vi "sub_PSKMod.vi"(0 "Packet to Transmit":i8[](array[numeric]), 2 "PSK system parameters":T2 {"PSK type" items=["normal", "shifted", "offset"]; "symbol map" format="%.3f"}, 7 "Symbol Rate, Hz":dbl=1.0 format="%.2f", 11 "error in (no error)":errorcluster, 12 "filter parameters":T1={"Alpha"=0.5, "Filter Length"=6, "TX Filter"=enum."Root Raised Cos"} {"Alpha" format="%.2f"}) -> (4 "output complex waveform":cluster{"t0":dbl, "dt":dbl, "Y":cdb[]} {"Y" format="%.3f"; "dt" format="%^.2e"; "t0" format="%.4f"}, 8 "samples per symbol":i32, 15 "error out":errorcluster)   [LabVIEW 2015]
uses:
  <vilib>/addons/Modulation/Analog/support/mod_Set Error Source.vi
  <vilib>/addons/Modulation/Digital/Support/Common/Validators/mod_Generate Filter Coefficients Validate.vi
  <vilib>/addons/Modulation/Digital/General/subVIs/mod_Generate Filter Coefficients.vi
  <vilib>/addons/Modulation/niDMT.lvlib
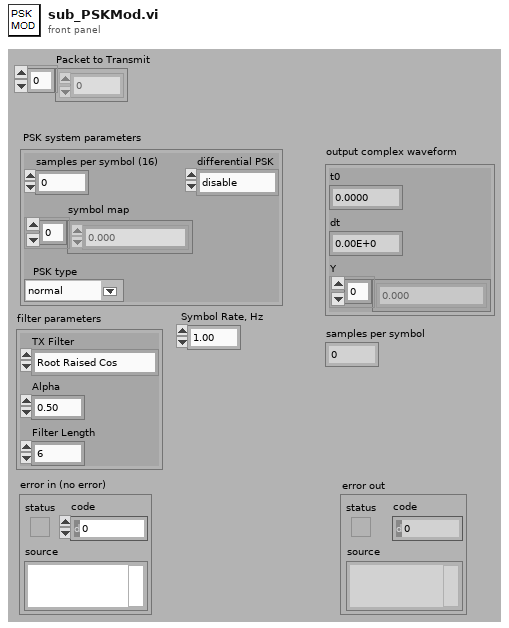
[diagram p1: front panel]
types:
  T1 = cluster{"Alpha":dbl, "Filter Length":i32, "TX Filter":enum16{"none", "Raised Cosine", "Root Raised Cos", "Gaussian"}}
  T2 = cluster{"samples per symbol (16)":i32, "symbol map":cdb[], "differential PSK":enum16{"disable", "enable"}, "PSK type":u16}
  T3 = enum16{"FSK", "PSK", "QAM", "MSK", "PAM", "ASK", "CPM"}
  T4 = enum16{"none", "Raised Cosine", "Root Raised Cos", "Gaussian"}
  T5 = typedef "niAMT.lvlib/Complex Data Waveform.ctl" = cluster{"t0":dbl, "dt":dbl, "Y":cdb[]}
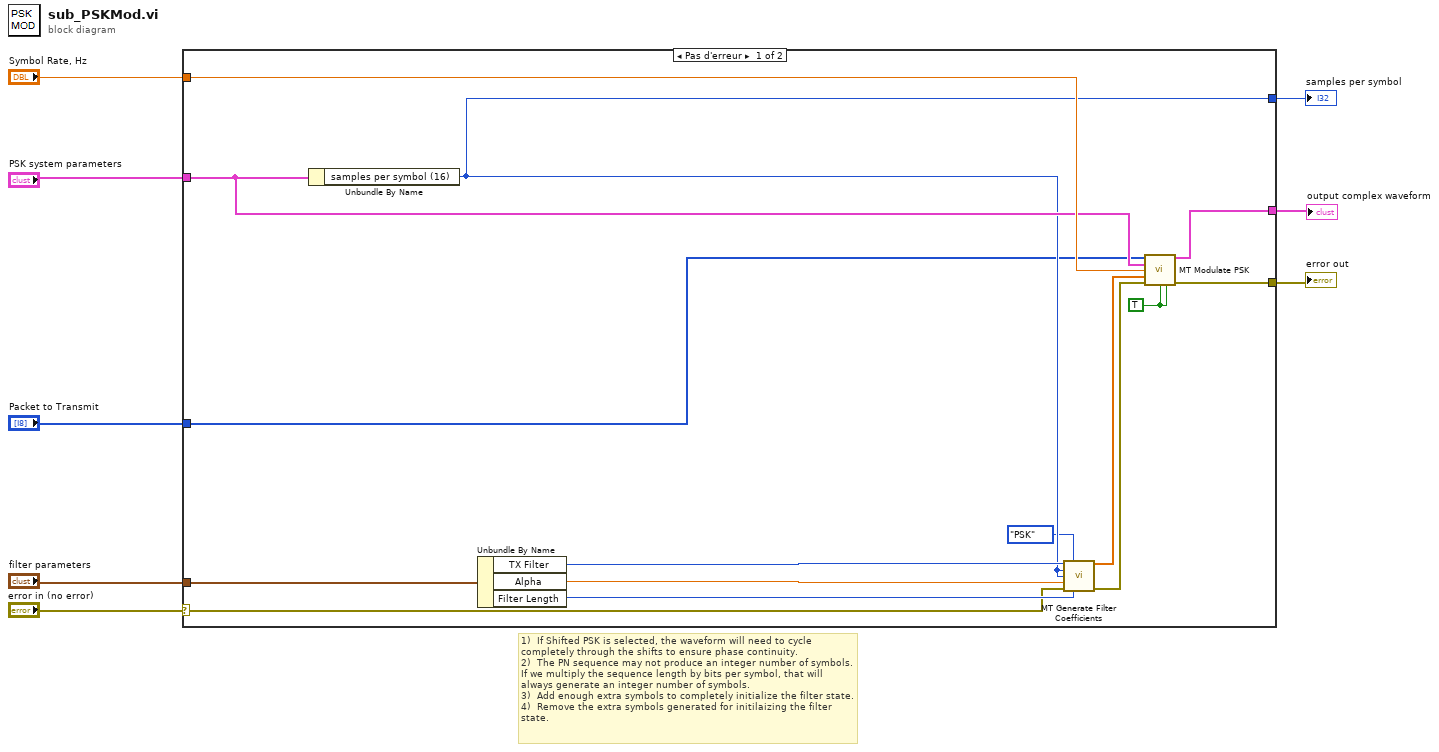
[diagram p0: block diagram]
diagram:
  # "1)  If Shifted PSK is selected, the waveform will need to cycle completely through the shifts to ensure phase continuity. \n2)  The PN sequence may not produce an integer number of symbols.  If we multiply the sequence length by bits per symbol, that will always generate an integer number of symbols. \n3)  Add enough extra symbols to completely initialize the filter state.\n4)  Remove the extra symbols generated for initilaizing the filter state."
  n1 = case shown="Pas d'erreur" "error in (no error)" {
    selector: "error in (no error)" -> [w10 w24]
    tunnel: [w15 _] -> w8
    tunnel: [w13 _] -> w7
    tunnel: [w23 w24] -> w6
    tunnel: "Symbol Rate, Hz" -> [w20 _]
    tunnel: "PSK system parameters" -> [w18 _]
    tunnel: "filter parameters" -> [w12 _]
    tunnel: "Packet to Transmit" -> [w14 _]
    frame No Error {
      w9 = TRUE ("Reset (T)")
      n2 = Unbundle By Name(w18) -> ("samples per symbol (16)"=w15:i32)
      n3 = Unbundle By Name(w12) -> ("TX Filter"=w21:T4, "Alpha"=w22:dbl, "Filter Length"=w17:i32)
      n4 = call <vilib>:"MT Generate Filter Coefficients.vi"("pulse shaping filter (none)"=w21, "modulation type"=T3."PSK", "pulse shaping samples per symbol (16)"=w15, "matched samples per symbol (16)"=w15, "filter parameter"=w22, "error in (no error)"=w10, "filter length (symbols)"=w17) -> ("pulse shaping filter coefficients"=w19:dbl[], "error out"=w16:errorcluster)  [unwired: 6 in, 1 out]
      n5 = call <vilib>:"MT Modulate PSK.vi"("input bit stream"=w14, "PSK system parameters"=w18, "symbol rate (Hz)"=w20, "pulse shaping filter coefficients"=w19, "error in (no error)"=w16, "reset? (T)"=w9, "flush buffers? (F)"=w9) -> ("output complex waveform"=w13:T5, "error out"=w23:errorcluster)  [unwired: 6 in, 1 out]
    }
    frame Error {
    }
  }
  "error out" <- w6
  "output complex waveform" <- w7
  "samples per symbol" <- w8
